vi "HeightMeasureUsingFocus.vi"(0 "controller in":refnum<k24>, 1 "StartZ":dbl, 5 "SessionIn":T2 caption="Session In", 7 "ImageIn":T1, 9 "ScanRange":dbl=0.4 format="%#_13g", 11 "error in (no error)":errorcluster, 12 "SafeZ":dbl) -> (3 "BestZ":dbl, 4 "controller out":refnum<k24>, 6 "Session Out":T2, 8 "Image Out":T1, 14 "MaxVal":dbl, 15 "Error Out":errorcluster)   [LabVIEW 2019]
uses:
  C:/Users/TTUHEP/Documents/LabVIEW/Other Models/2010/Bin/Aerotech.A3200.dll
  Other Models/2010/Bin/Aerotech.A3200.dll
  <vilib>/userDefined/High Color/IMAQdx.ctl
  <vilib>/vision/Image Controls.llb/IMAQ Image.ctl
panel:
  in  "InitialStepSize":dbl=0.1
  in  "StopScan":bool
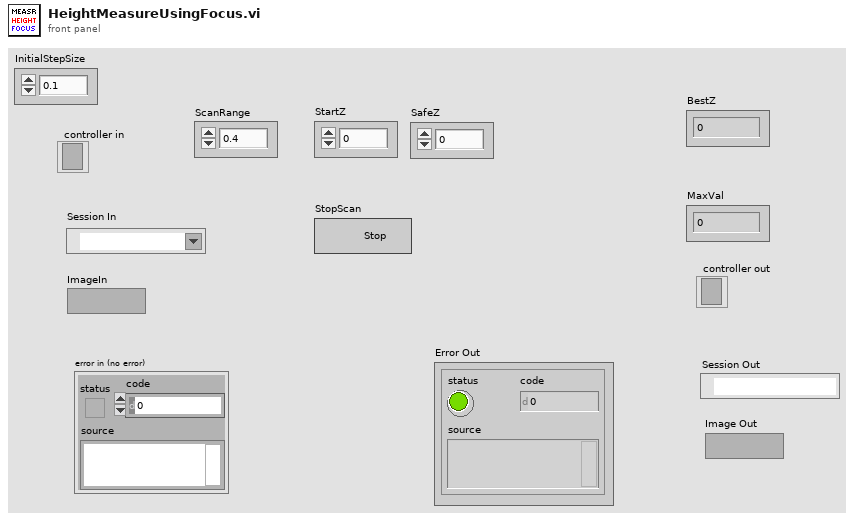
[diagram p1: front panel]
types:
  T1 = typedef "IMAQ Image.ctl" = refnum<image>
  T2 = typedef "IMAQdx.ctl" = refnum<k21>
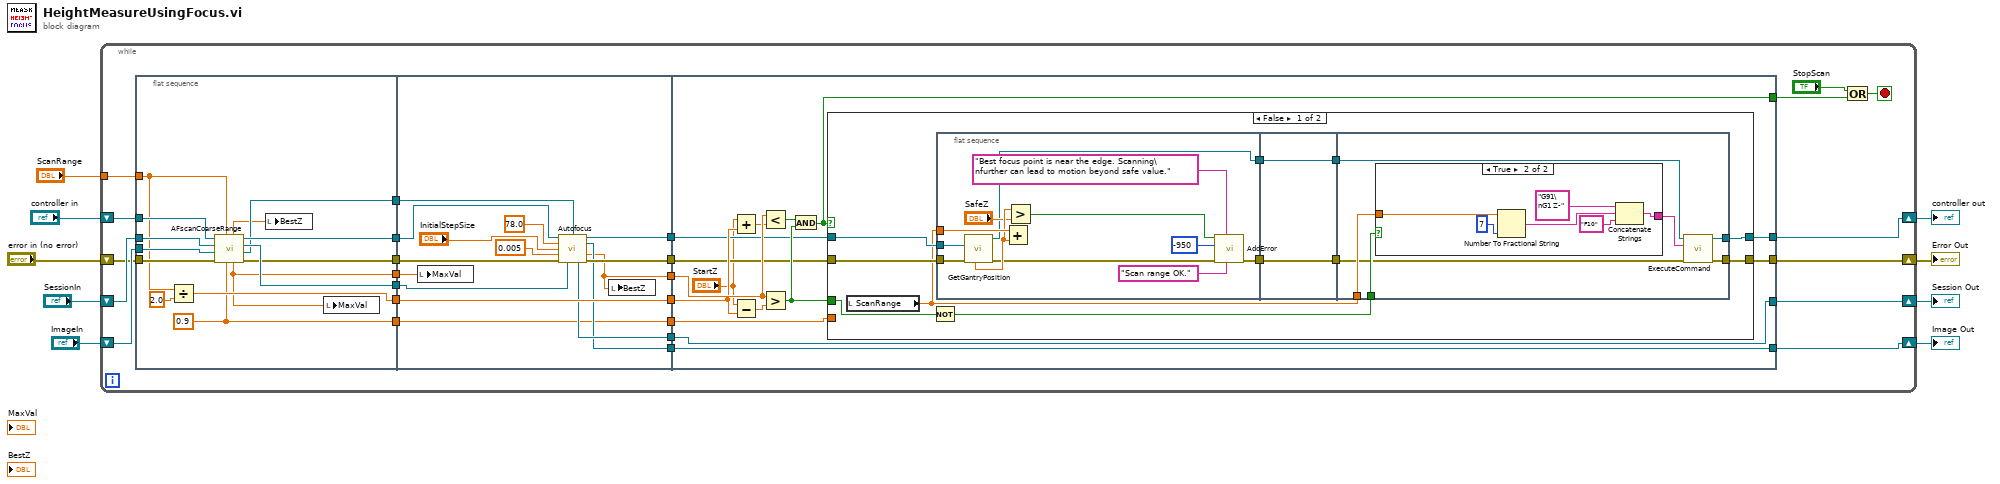
[diagram p0: block diagram]
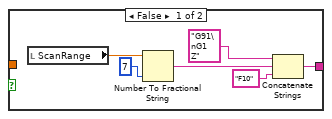
[diagram p2: hidden frame]
diagram:
  n1 = while {
    tunnel: "ScanRange" -> [w20]
    shift-right: [w19] -> w3
    shift-left: "controller in" -> [w14]
    shift-right: [w18] -> w4
    shift-left: "error in (no error)" -> [w13]
    shift-right: [w12] -> w1
    shift-left: "SessionIn" -> [w22]
    shift-right: [w11] -> w2
    shift-left: "ImageIn" -> [w21]
    stop <- w16 stop-if-true
    n2 = flat-sequence {
      tunnel: w14 -> [w49]
      tunnel: w22 -> [w48]
      tunnel: w21 -> [w47]
      tunnel: w13 -> [w46]
      tunnel: [w45] -> w35
      tunnel: [w44] -> w34
      tunnel: [w43] -> w33
      tunnel: [w42] -> w32
      tunnel: [w40] -> w31
      tunnel: [w39] -> w30
      tunnel: w20 -> [w38]
      tunnel: [w36] -> w10
      tunnel: w35 -> [w61]
      tunnel: w34 -> [w62]
      tunnel: w33 -> [w63]
      tunnel: w32 -> [w64]
      tunnel: [w51] -> w29
      tunnel: w31 -> [w60]
      tunnel: [w60] -> w28
      tunnel: [w59] -> w27
      tunnel: [w58] -> w26
      tunnel: [w57] -> w25
      tunnel: [w56] -> w24
      tunnel: [w55] -> w23
      tunnel: w30 -> [w55]
      tunnel: w10 -> [w50]
      tunnel: w29 -> [w78]
      tunnel: w28 -> [w77]
      tunnel: w27 -> [w73]
      tunnel: w26 -> [w72]
      tunnel: w25 -> [w66]
      tunnel: w24 -> [w65]
      tunnel: w23 -> [w70]
      tunnel: [w69] -> w15
      tunnel: [w68] -> w19
      tunnel: [w67] -> w18
      tunnel: [w66] -> w12
      tunnel: [w65] -> w11
      frame #0 {
        w39 = 0.9 ("StopAfterMaxFrac")
        n3 = Divide(x=w38, y=2.0) -> (x/y=w40:dbl)
        n4 = call "AFscanCoarseRange.vi"("StopAfterMaxFrac"=w39, "ScanRange"=w38, "error in (no error)"=w46, "ImageIn"=w47, "SessionIn"=w48, "controller in"=w49) -> ("error out"=w42:errorcluster, "Image Out"=w43:T1, "Session Out"=w44:T2, "controller out"=w45:refnum<k24>, "MaxVal"=w36:dbl, "BestZ"=w37:dbl)
        n5 = local write "BestZ"(w37) -> ()
        n6 = local write "MaxVal"(w36) -> ()
      }
      frame #1 {
        n7 = local write "MaxVal"(w50) -> ()
        n8 = call "Autofocus.vi"("controller in"=w61, "ImageIn"=w63, "SafeMaxZ"=78.0, "InitialStepSize"="InitialStepSize", "Tolerance"=0.005, "error in (no error)"=w64, "SessionIn"=w62) -> ("controller out"=w59:refnum<k24>, "Image"=w56:T1, "BestZvalue"=w51:dbl, "Session Out"=w57:T2, "error out"=w58:errorcluster)  [unwired: 3 in, 1 out]
        n9 = local write "BestZ"(w51) -> ()
      }
      frame #2 {
        n10 = Add(x="StartZ", y=w77) -> (x+y=w76:dbl)
        n11 = Subtract(x="StartZ", y=w77) -> (x-y=w79:dbl)
        n12 = Less?(x=w78, y=w76) -> (x < y?=w75:bool)
        n13 = Greater?(x=w78, y=w79) -> (0:w74:bool)
        n14 = And(x=w75, y=w74) -> (x .and. y?=w69:bool)
        n15 = case shown="False" w69 {
          tunnel: w74 -> [w90 _]
          tunnel: w73 -> [w89 w125]
          tunnel: w72 -> [w88 w124]
          tunnel: w70 -> [_ _]
          tunnel: [w81 w125] -> w68
          tunnel: [w80 w124] -> w67
          frame False {
            n16 = local read "ScanRange"() -> (w86:dbl)
            n17 = Not(x=w90) -> (.not. x?=w87:bool)
            n18 = flat-sequence {
              tunnel: w86 -> [w102]
              tunnel: w89 -> [w101]
              tunnel: w88 -> [w100]
              tunnel: [w92] -> w85
              tunnel: [w91] -> w83
              tunnel: w85 -> [w104]
              tunnel: [w104] -> w84
              tunnel: w83 -> [w103]
              tunnel: [w103] -> w82
              tunnel: w87 -> [w111]
              tunnel: w86 -> [w110]
              tunnel: w84 -> [w108]
              tunnel: w82 -> [w107]
              tunnel: [w106] -> w81
              tunnel: [w105] -> w80
              frame #0 {
                n19 = call "GetGantryPosition.vi"("error in (no error)"=w100, "Controller In"=w101) -> ("error out"=w94:errorcluster, "controller out"=w91:refnum<k24>, "Position Z"=w99:dbl)  [unwired: 3 in, 4 out]
                n20 = Add(x=w102, y=w99) -> ()  [unwired: 1 out]
                n21 = Greater?(x=w99, y="SafeZ") -> (0:w97:bool)
                n22 = call "AddError.vi"("NoErrorMessage"="Scan range OK.", "ErrorMessage"="Best focus point is near the edge. Scanning\nfurther can lead to motion beyond safe value.", "error in"=w94, "code"=-950, "Error?"=w97) -> ("Error out"=w92:errorcluster)  [unwired: 6 in]
              }
              frame #1 {
              }
              frame #2 {
                n23 = case shown="True" w111 {
                  tunnel: [w112 w119] -> w109
                  tunnel: w110 -> [_ w118]
                  frame False {
                    n24 = local read "ScanRange"() -> (w113:dbl)
                    n25 = Number To Fractional String(number=w113, precision (6)=i16 7) -> (F-format string=w114:string)  [unwired: 2 in]
                    n26 = Concatenate Strings("G91\nG1 Z", w114, "F10" ("string")) -> (w112:string)
                  }
                  frame True {
                    n27 = Number To Fractional String(number=w118, precision (6)=i16 7) -> (F-format string=w120:string)  [unwired: 2 in]
                    n28 = Concatenate Strings("G91\nG1 Z-", w120, "F10" ("string")) -> (w119:string)
                  }
                }
                n29 = call "ExecuteCommand.vi"("error in (no error)"=w108, "Command Code"=w109, "controller in"=w107) -> ("error out"=w105:errorcluster, "controller out"=w106:refnum<k24>)  [unwired: 6 in, 1 out]
              }
            }
          }
          frame True {
          }
        }
      }
    }
    n30 = Or(x="StopScan", y=w15) -> (x .or. y?=w16:bool)
  }
  "Error Out" <- w4
  "controller out" <- w3
  "Image Out" <- w2
  "Session Out" <- w1
